vi "lectura_simultanea.vi"(10 "Address Type":T1=1 items=["Public", "Random"], 11 "COM Bluegiga in":refnum<visa-resource-name>="COM13") -> (3 "Connected":bool)   [LabVIEW 2020]
uses:
  <vilib>/BLE/type_def/connection_status_bundle.ctl
  <vilib>/BLE/type_def/address_type.ctl
panel:
  in  "stop":bool
  out "Text":string caption="Result"
  out "Numeric":dbl
  out "w 2":dbl
  out "x 2":dbl
  out "y 2":dbl
  out "z 2":dbl
  out "MAC Address":string
  out "Handle table":string[][](array[string])
  out "Connection Status":T2={"MAC Address"="", "cnx handle"=0, "cnx flags"=0, "Address Type"=125, "Connection Interval (ms)"=125, "Timeout(ms)"=125, "Latency"=0, "bonding handle"=0} {"Address Type" items=["Public", "Random"]}
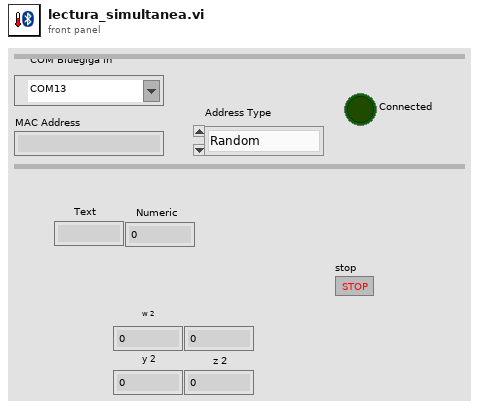
[diagram p1: front panel]
types:
  T1 = typedef "address_type.ctl" = u8
  T2 = typedef "connection_status_bundle.ctl" = cluster{"MAC Address":string, "cnx handle":u8, "cnx flags":u8, "Address Type":T1, "Connection Interval (ms)":u16, "Timeout(ms)":u16, "Latency":u16, "bonding handle":u8}
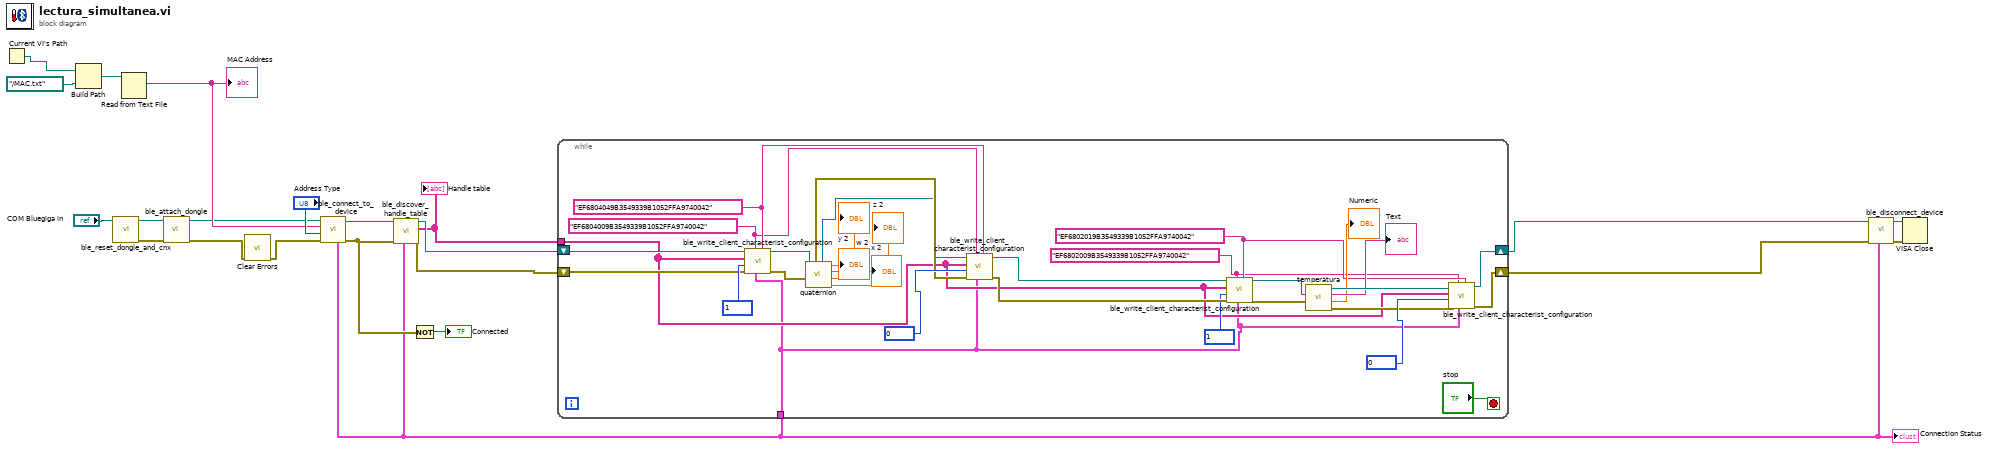
[diagram p0: block diagram]
diagram:
  n1 = Current VI's Path() -> (path=w10:path)
  n2 = Build Path(base path=w10, name or relative path=path "../MAC.txt") -> (appended path=w11:path)
  n3 = call <vilib>:"ble_reset_dongle_and_cnx.vi"("COM Bluegiga in"="COM Bluegiga in") -> ("error out"=w20:errorcluster, "COM Bluegiga out"=w18:refnum<visa-resource-name>)  [unwired: 9 in]
  n4 = Read from Text File(file (use dialog)=w11) -> (text=w13:string)  [unwired: 3 in, 3 out]
  "MAC Address" <- w13
  n5 = call <vilib>:"ble_attach_dongle.vi"("error in (no error)"=w20, "COM Bluegiga in"=w18) -> ("error out"=w8:errorcluster, "COM Bluegiga out"=w9:refnum<visa-resource-name>)  [unwired: 8 in]
  n6 = call <vilib>:"Clear Errors.vi"("error in (no error)"=w8) -> ("error out"=w15:errorcluster)  [unwired: 5 in, 1 out]
  n7 = call <vilib>:"ble_connect_to_device.vi"("Address Type"="Address Type", "error in (no error)"=w15, "MAC Address"=w13, "COM Bluegiga in"=w9) -> ("error out"=w16:errorcluster, "COM Bluegiga out"=w17:refnum<visa-resource-name>, "Connection Status"=w1:T2)  [unwired: 5 in]
  "Connection Status" <- w1
  n8 = call <vilib>:"ble_discover_handle_table.vi"("Connection Status"=w1, "error in (no error)"=w16, "COM Bluegiga in"=w17) -> ("error out"=w5:errorcluster, "Handle table"=w2:string[][], "COM Bluegiga out"=w6:refnum<visa-resource-name>)  [unwired: 6 in]
  "Handle table" <- w2
  n9 = Not(x=w16) -> (.not. x?=→"Connected":bool)
  n10 = while {
    shift-right: [w32] -> w4
    shift-left: w6 -> [w33]
    shift-right: [w30] -> w3
    shift-left: w5 -> [w31]
    tunnel: w2 -> [w24]
    tunnel: w1 -> [w23]
    stop <- "stop" stop-if-true
    w27 = "EF6802019B3549339B1052FFA9740042" ("Characteristic UUID")
    w26 = "EF6802009B3549339B1052FFA9740042" ("Service UUID")
    w29 = "EF6804049B3549339B1052FFA9740042" ("Characteristic UUID")
    w28 = "EF6804009B3549339B1052FFA9740042" ("Service UUID")
    n11 = call <vilib>:"ble_write_client_characterist_configuration.vi"("Characteristic UUID"=w29, "Connection Status"=w23, "Service UUID"=w28, "error in (no error)"=w31, "Value(16bit)"=u16 1, "Handle table"=w24, "COM Bluegiga in"=w33) -> ("error out"=w44:errorcluster, "COM Bluegiga out"=w45:refnum<visa-resource-name>)  [unwired: 3 in]
    n12 = call "quaternion.vi"("error in (no error)"=w44, "COM Bluegiga in"=w45) -> ("z"=→"z 2":dbl, "y"=→"y 2":dbl, "x"=→"x 2":dbl, "w"=→"w 2":dbl, "COM Bluegiga out"=w42:refnum<visa-resource-name>, "error out"=w43:errorcluster)  [unwired: 4 in]
    n13 = call <vilib>:"ble_write_client_characterist_configuration.vi"("Characteristic UUID"=w29, "Connection Status"=w23, "Service UUID"=w28, "error in (no error)"=w43, "Value(16bit)"=u16 0, "Handle table"=w24, "COM Bluegiga in"=w42) -> ("error out"=w52:errorcluster, "COM Bluegiga out"=w53:refnum<visa-resource-name>)  [unwired: 3 in]
    n14 = call <vilib>:"ble_write_client_characterist_configuration.vi"("Characteristic UUID"=w27, "Connection Status"=w23, "Service UUID"=w26, "error in (no error)"=w52, "Value(16bit)"=u16 1, "Handle table"=w24, "COM Bluegiga in"=w53) -> ("error out"=w38:errorcluster, "COM Bluegiga out"=w39:refnum<visa-resource-name>)  [unwired: 3 in]
    n15 = call "temperatura.vi"("error in (no error)"=w38, "COM Bluegiga in"=w39) -> ("error out"=w36:errorcluster, "Numeric"=→"Numeric":dbl, "Text"=→"Text":string, "COM Bluegiga out"=w37:refnum<visa-resource-name>)  [unwired: 6 in]
    n16 = call <vilib>:"ble_write_client_characterist_configuration.vi"("Characteristic UUID"=w27, "Connection Status"=w23, "Service UUID"=w26, "error in (no error)"=w36, "Value(16bit)"=u16 0, "Handle table"=w24, "COM Bluegiga in"=w37) -> ("error out"=w30:errorcluster, "COM Bluegiga out"=w32:refnum<visa-resource-name>)  [unwired: 3 in]
  }
  n17 = call <vilib>:"ble_disconnect_device.vi"("Connection Status"=w1, "error in (no error)"=w3, "COM Bluegiga in"=w4) -> ("error out"=w21:errorcluster, "COM Bluegiga out"=w22:refnum<visa-resource-name>)  [unwired: 7 in]
  n18 = VISA Close(VISA resource name=w22, error in (no error)=w21) -> ()  [unwired: 1 out]
